vi "niDTS BT Tx Test UTIL Static Default Parameters.vi"(9 "ModulationCharacter Select":T1=enum."BOTH", 10 "BT Standard":T2 caption="802.11 Standard") -> (2 "BT Tx Input Parameters":T3={"Channel"=0, "Data Rate "=1, "Dut Tx Power"=0.0, "External Attenuation (dB)"=[0.0, 0.0, 0.0, 0.0], "Auto Level"=FALSE, "Packet type"=enum."DH1", "Payload Pattern"=enum."PN9", "Burst Sync"=enum."PREamble", "BD ADDRESS"=0, "Packet Length, bytes"=37, "ModAcc Measurement Paramaters"={"ModAcc Enable"=FALSE, "CFO Enable"=FALSE, "Character Select"=enum."DF1", "Averages"=1, "Averaging Mode"=enum."RMS", "Measurement Length"=-1, "Measurement Offset"=0}, "OBW Measurement Parameters"={"OBW Enable"=FALSE, "OBW Averages"=1, "Averaging Type"=enum."RMS", "Measurement Interval Mode"=enum."AUTO", "Measurement Interval Length (sec)"=0.005}, "TXP Measurement Parameters"={"TXP Power Enable"=FALSE, "TXP Averages"=1, "Averaging Type"=enum."RMS"}, "IBE  Measurement Parameters"={"IBE Enable"=FALSE, "IBE Averages"=1, "Averaging Type"=enum."RMS", "Numbe of Channels"=11, "Channel Mode"=enum."Centered", "Measurement Interval Mode"=enum."AUTO", "Measurement Interval Length (sec)"=0.005}, "Trace Enable"=FALSE, "Trigger"={"MinQuietTimeDuration (sec)"=0.0001, "TriggerDelay (sec)"=0.0, "TriggerEdge"=enum."RISing", "TriggerSource"=enum."RF0", "TriggerThreshold (dB)"=-20.0, "TriggerTimeout (sec)"=10.0}} {"BD ADDRESS" max=16777215 format="%.0x"})   [LabVIEW 2015, in "niDTS BT.lvlib"]
uses:
  niDTS BT.lvlib
  Includes/niDTS BT Tx Test INC Parameters.ctl
  Includes/niDTS BT INC Packet Type.ctl
  Includes/niDTS BT Tx Test INC BD Payload Data.ctl
  Includes/niDTS BT Tx Test INC Modulation Characteristics.ctl
  Includes/niDTS BT INC OBW Measurement Parameters.ctl
  Includes/niDTS BT INC TXP Measurement Parameters.ctl
  EDR Tx Test/Includes/niDTS BT INC EDR IBE Measurement Parameters.ctl
  Includes/niDTS BT DUT INC Trigger.ctl
  Includes/niDTS BT INC Standard.ctl
  BDR Tx Test/Includes/niDTS BT BDR Tx Test INC Parameters.ctl
  BDR Tx Test/Includes/niDTS BT INC BDR Packet Type.ctl
  BDR Tx Test/Includes/niDTS BT INC BDR ACP Measurement Parameters.ctl
  EDR Tx Test/Includes/niDTS BT EDR Tx Test INC Parameters.ctl
  EDR Tx Test/Includes/niDTS BT INC EDR Packet Type.ctl
  EDR Tx Test/Includes/niDTS BT INC EDR Data Rate.ctl
  EDR Tx Test/Includes/niDTS BT INC EDR Burst Sync.ctl
  EDR Tx Test/Includes/niDTS BT INC EDR ModAcc Measurement Parameters.ctl
  LE Tx Test/Includes/niDTS BT LE Tx Test INC Parameters.ctl
  LE Tx Test/Includes/niDTS BT INC LE IBE Measurement Parameters.ctl
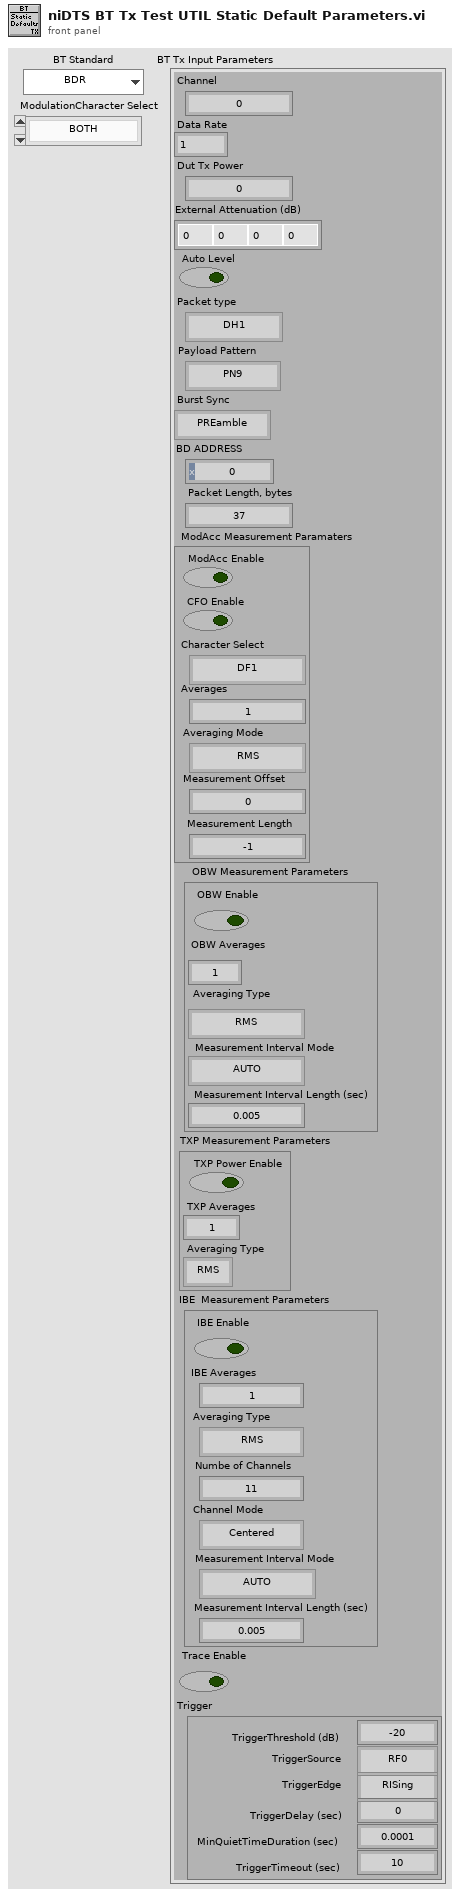
[diagram p1: front panel]
types:
  T1 = typedef "niDTS BT.lvlib/niDTS BT Tx Test INC Modulation Characteristics.ctl" = enum16{"DF1", "DF2", "BOTH"}
  T2 = typedef "niDTS BT.lvlib/niDTS BT INC Standard.ctl" = enum16{"BDR", "EDR", "LE-TP"}
  T3 = typedef "niDTS BT.lvlib/niDTS BT Tx Test INC Parameters.ctl" = cluster{"Channel":i32, "Data Rate ":i32, "Dut Tx Power":dbl, "External Attenuation (dB)":dbl[], "Auto Level":bool, "Packet type":T4, "Payload Pattern":T5, "Burst Sync":enum16{"NONE", "PREamble"}, "BD ADDRESS":u32, "Packet Length, bytes":i32, "ModAcc Measurement Paramaters":cluster{"ModAcc Enable":bool, "CFO Enable":bool, "Character Select":T1, "Averages":i32, "Averaging Mode":enum16{"RMS", "LOG", "SCALAR", "MAX", "MIN", "VECTOR"}, "Measurement Length":i32, "Measurement Offset":i32}, "OBW Measurement Parameters":T6, "TXP Measurement Parameters":T7, "IBE  Measurement Parameters":T8, "Trace Enable":bool, "Trigger":T9}
  T4 = typedef "niDTS BT.lvlib/niDTS BT INC Packet Type.ctl" = enum16{"NULL", "POLL", "FHS", "DM1", "DH1", "HV1", "HV2", "HV3", "EV3", "DV", "AUX1", "DM3", "DH3", "EV4", "EV5", "DM5", "DH5", "LE-TP"}
  T5 = typedef "niDTS BT.lvlib/niDTS BT Tx Test INC BD Payload Data.ctl" = enum16{"0", "1", "01", "00001111", "PN9", "AUTO"}
  T6 = typedef "niDTS BT.lvlib/niDTS BT INC OBW Measurement Parameters.ctl" = cluster{"OBW Enable":bool, "OBW Averages":i32, "Averaging Type":enum16{"RMS", "LOG", "SCALAR", "MAX", "MIN", "VECTOR"}, "Measurement Interval Mode":enum16{"AUTO", "MANUAL"}, "Measurement Interval Length (sec)":dbl}
  T7 = typedef "niDTS BT.lvlib/niDTS BT INC TXP Measurement Parameters.ctl" = cluster{"TXP Power Enable":bool, "TXP Averages":i32, "Averaging Type":enum16{"RMS", "LOG", "SCALAR", "MAX", "MIN"}}
  T8 = typedef "niDTS BT.lvlib/niDTS BT INC EDR IBE Measurement Parameters.ctl" = cluster{"IBE Enable":bool, "IBE Averages":i32, "Averaging Type":enum16{"RMS", "LOG", "SCALAR", "MAX", "MIN", "VECTOR"}, "Numbe of Channels":i32, "Channel Mode":enum16{"InBand", "Centered"}, "Measurement Interval Mode":enum16{"AUTO", "MANUAL"}, "Measurement Interval Length (sec)":dbl}
  T9 = typedef "niDTS BT.lvlib/niDTS BT DUT INC Trigger.ctl" = cluster{"MinQuietTimeDuration (sec)":dbl, "TriggerDelay (sec)":dbl, "TriggerEdge":enum16{"RISing", "FALLing"}, "TriggerSource":enum16{"IMMediate", "RF0", "PFI0", "PFI1", "RTS0", "RTS1", "RTS2", "RTS3", "RTS4", "RTS5", "RTS6", "RTS7", "PXIStar", "SOFT"}, "TriggerThreshold (dB)":dbl, "TriggerTimeout (sec)":dbl}
  T10 = typedef "niDTS BT.lvlib/niDTS BT BDR Tx Test INC Parameters.ctl" = cluster{"Channel":i32, "Dut Tx Power (dBm)":dbl, "Auto Level":bool, "External Attenuation (dB)":dbl, "BDR Packet type":T11, "Payload Data":T5, "Burst Sync":enum16{"NONE", "PREamble"}, "Packet length (bytes)":i32, "BD ADDRESS":string, "Modulation Measurement":cluster{"ModAcc Enable":bool, "CFO Enable":bool, "Character Select":T1, "Averages":i32, "Averaging Mode":enum16{"RMS", "LOG", "SCALAR", "MAX", "MIN", "VECTOR"}, "Measurement Duration (Symbols)":i32, "Measurement Offset (Symbols)":i32}, "Trace Enable":bool, "OBW Measurement":T6, "TXP Measurement":T7, "IBE Measurement":T12, "Trigger":T9}
  T11 = typedef "niDTS BT.lvlib/niDTS BT INC BDR Packet Type.ctl" = enum16{"NULL", "POLL", "FHS", "DM1", "DH1", "HV1", "HV2", "HV3", "EV3", "DV", "AUX1", "DM3", "DH3", "EV4", "EV5", "DM5", "DH5"}
  T12 = typedef "niDTS BT.lvlib/niDTS BT INC BDR ACP Measurement Parameters.ctl" = cluster{"IBE Enable":bool, "IBE Averages":i32, "Averaging Type":enum16{"RMS", "LOG", "SCALAR", "MAX", "MIN", "VECTOR"}, "Numbe of Channels":i32, "Channel Mode":enum16{"InBand", "Centered"}, "Measurement Interval Mode":enum16{"AUTO", "MANUAL"}, "Measurement Interval Length (sec)":dbl}
  T13 = typedef "niDTS BT.lvlib/niDTS BT EDR Tx Test INC Parameters.ctl" = cluster{"Channel":i32, "Dut Tx Power  (dBm)":dbl, "Auto Level":bool, "External Attenuation (dB)":dbl, "EDR Packet type":T14, "Data Rate":T15, "Payload Data":T5, "Burst Sync":T16, "Packet Length, bytes":i32, "BD ADDRESS":string, "Trace Enable":bool, "EDR ModAcc Measurement":T17, "TXP Measurement":T7, "IBE  Measurement":T8, "Trigger":T9}
  T14 = typedef "niDTS BT.lvlib/niDTS BT INC EDR Packet Type.ctl" = enum16{"NULL", "POLL", "FHS", "DM1", "DH1", "HV1", "HV2", "HV3", "EV3", "DV", "AUX1", "DM3", "DH3", "EV4", "EV5", "DM5", "DH5"}
  T15 = typedef "niDTS BT.lvlib/niDTS BT INC EDR Data Rate.ctl" = i32
  T16 = typedef "niDTS BT.lvlib/niDTS BT INC EDR Burst Sync.ctl" = enum16{"NONE", "PREamble"}
  T17 = typedef "niDTS BT.lvlib/niDTS BT INC EDR ModAcc Measurement Parameters.ctl" = cluster{"DEVM Enable":bool, "Averages":i32, "Averaging Mode":enum16{"RMS", "LOG", "SCALAR", "MAX", "MIN", "VECTOR"}, "Measurement Duration (bytes)":i32, "Measurement Offset (bytes)":i32}
  T18 = typedef "niDTS BT.lvlib/niDTS BT LE Tx Test INC Parameters.ctl" = cluster{"Channel":i32, "Dut Tx Power (dBm)":dbl, "Auto Level":bool, "External Attenuation (dB)":dbl, "Payload Data":T5, "Burst Sync":enum16{"NONE", "PREamble"}, "Packet Length (bytes)":i32, "Modulation Measurement":cluster{"ModAcc Enable":bool, "CFO Enable":bool, "Character Select":T1, "Averages":i32, "Averaging Mode":enum16{"RMS", "LOG", "SCALAR", "MAX", "MIN", "VECTOR"}, "Measurement Duration (bytes)":i32, "Measurement Offset (bytes)":i32}, "TXP Measurement":T7, "LE IBE Measurement":T19, "Trace Enable":bool, "Trigger":T9}
  T19 = typedef "niDTS BT.lvlib/niDTS BT INC LE IBE Measurement Parameters.ctl" = cluster{"LE IBE Enable":bool, "LE IBE Averages":i32, "Averaging Type":enum16{"RMS", "LOG", "SCALAR", "MAX", "MIN", "VECTOR"}, "Numbe of Channels":i32, "Channel Mode":enum16{"InBand", "Centered"}, "Measurement Interval Mode":enum16{"AUTO", "MANUAL"}, "Measurement Interval Length (sec)":dbl}
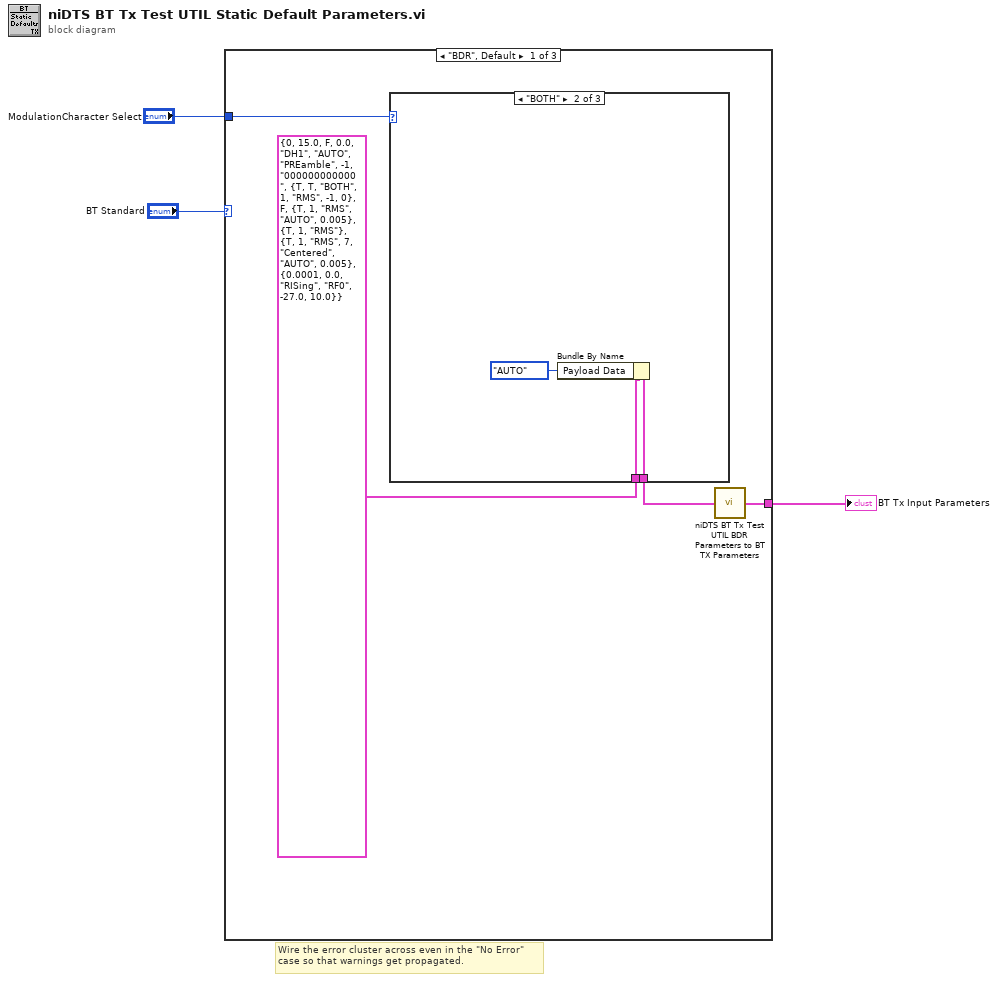
[diagram p0: block diagram]
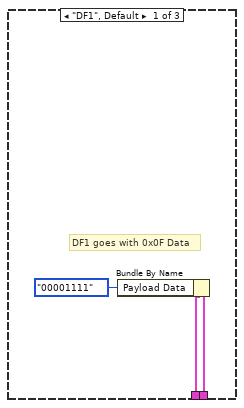
[diagram p2: hidden frame]
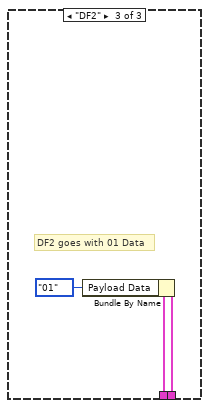
[diagram p3: hidden frame]
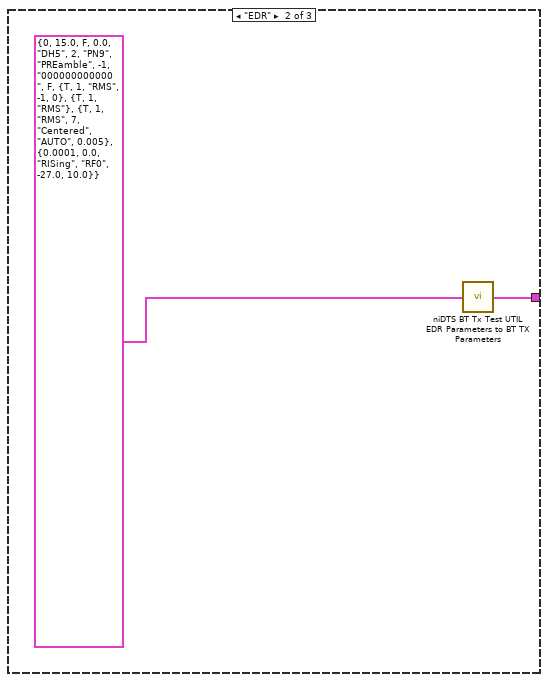
[diagram p4: hidden frame]
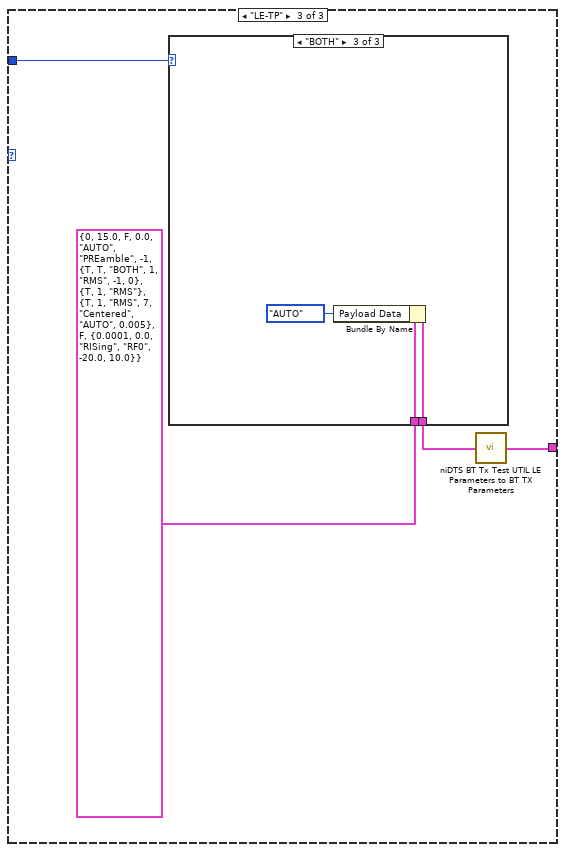
[diagram p5: hidden frame]
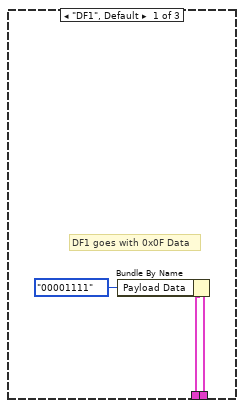
[diagram p6: hidden frame]
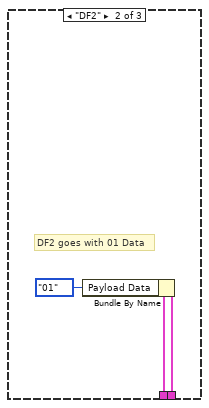
[diagram p7: hidden frame]
diagram:
  # "Wire the error cluster across even in the \"No Error\"\ncase so that warnings get propagated."
  n1 = case shown="\"BDR\", Default" "BT Standard" {
    tunnel: [w7 w18 w22] -> w2
    tunnel: "ModulationCharacter Select" -> [w4 _ w21]
    frame "BDR", Default {
      n2 = case shown="\"BOTH\"" w4 {
        tunnel: T10 {"Channel"=0, "Dut Tx Power (dBm)"=15.0, "Auto Level"=FALSE, "External Attenuation (dB)"=0.0, "BDR Packet type"=enum."DH1", "Payload Data"=enum."AUTO", "Burst Sync"=enum."PREamble", "Packet length (bytes)"=-1, "BD ADDRESS"="000000000000 ", "Modulation Measurement"={"ModAcc Enable"=TRUE, "CFO Enable"=TRUE, "Character Select"=enum."BOTH", "Averages"=1, "Averaging Mode"=enum."RMS", "Measurement Duration (Symbols)"=-1, "Measurement Offset (Symbols)"=0}, "Trace Enable"=FALSE, "OBW Measurement"={"OBW Enable"=TRUE, "OBW Averages"=1, "Averaging Type"=enum."RMS", "Measurement Interval Mode"=enum."AUTO", "Measurement Interval Length (sec)"=0.005}, "TXP Measurement"={"TXP Power Enable"=TRUE, "TXP Averages"=1, "Averaging Type"=enum."RMS"}, "IBE Measurement"={"IBE Enable"=TRUE, "IBE Averages"=1, "Averaging Type"=enum."RMS", "Numbe of Channels"=7, "Channel Mode"=enum."Centered", "Measurement Interval Mode"=enum."AUTO", "Measurement Interval Length (sec)"=0.005}, "Trigger"={"MinQuietTimeDuration (sec)"=0.0001, "TriggerDelay (sec)"=0.0, "TriggerEdge"=enum."RISing", "TriggerSource"=enum."RF0", "TriggerThreshold (dB)"=-27.0, "TriggerTimeout (sec)"=10.0}} ("BDR Tx Input Parameters") -> [w9 w12 w16]
        tunnel: [w8 w11 w15] -> w5
        frame "DF1", Default {
          # "DF1 goes with 0x0F Data"
          n3 = Bundle By Name(cluster=w9, "Payload Data"=niDTS_BT_Tx_Test_INC_BD_Payload_Data."00001111") -> (w8:T10)
        }
        frame "BOTH" {
          n4 = Bundle By Name(cluster=w12, "Payload Data"=niDTS_BT_Tx_Test_INC_BD_Payload_Data."AUTO") -> (w11:T10)
        }
        frame "DF2" {
          # "DF2 goes with 01 Data"
          n5 = Bundle By Name(cluster=w16, "Payload Data"=niDTS_BT_Tx_Test_INC_BD_Payload_Data."01") -> (w15:T10)
        }
      }
      n6 = call "niDTS BT Tx Test UTIL BDR Parameters to BT TX Parameters.vi"("BT BDR Parameters"=w5) -> ("BT Tx Parameters"=w7:T3)  [unwired: 14 in]
    }
    frame "EDR" {
      n7 = call "niDTS BT Tx Test UTIL EDR Parameters to BT TX Parameters.vi"("EDR Tx Input Parameters"=T13 {"Channel"=0, "Dut Tx Power  (dBm)"=15.0, "Auto Level"=FALSE, "External Attenuation (dB)"=0.0, "EDR Packet type"=enum."DH5", "Data Rate"=2, "Payload Data"=enum."PN9", "Burst Sync"=enum."PREamble", "Packet Length, bytes"=-1, "BD ADDRESS"="000000000000 ", "Trace Enable"=FALSE, "EDR ModAcc Measurement"={"DEVM Enable"=TRUE, "Averages"=1, "Averaging Mode"=enum."RMS", "Measurement Duration (bytes)"=-1, "Measurement Offset (bytes)"=0}, "TXP Measurement"={"TXP Power Enable"=TRUE, "TXP Averages"=1, "Averaging Type"=enum."RMS"}, "IBE  Measurement"={"IBE Enable"=TRUE, "IBE Averages"=1, "Averaging Type"=enum."RMS", "Numbe of Channels"=7, "Channel Mode"=enum."Centered", "Measurement Interval Mode"=enum."AUTO", "Measurement Interval Length (sec)"=0.005}, "Trigger"={"MinQuietTimeDuration (sec)"=0.0001, "TriggerDelay (sec)"=0.0, "TriggerEdge"=enum."RISing", "TriggerSource"=enum."RF0", "TriggerThreshold (dB)"=-27.0, "TriggerTimeout (sec)"=10.0}}) -> ("BT Tx Input Parameters"=w18:T3)  [unwired: 14 in]
    }
    frame "LE-TP" {
      n8 = case shown="\"BOTH\"" w21 {
        tunnel: T18 {"Channel"=0, "Dut Tx Power (dBm)"=15.0, "Auto Level"=FALSE, "External Attenuation (dB)"=0.0, "Payload Data"=enum."AUTO", "Burst Sync"=enum."PREamble", "Packet Length (bytes)"=-1, "Modulation Measurement"={"ModAcc Enable"=TRUE, "CFO Enable"=TRUE, "Character Select"=enum."BOTH", "Averages"=1, "Averaging Mode"=enum."RMS", "Measurement Duration (bytes)"=-1, "Measurement Offset (bytes)"=0}, "TXP Measurement"={"TXP Power Enable"=TRUE, "TXP Averages"=1, "Averaging Type"=enum."RMS"}, "LE IBE Measurement"={"LE IBE Enable"=TRUE, "LE IBE Averages"=1, "Averaging Type"=enum."RMS", "Numbe of Channels"=7, "Channel Mode"=enum."Centered", "Measurement Interval Mode"=enum."AUTO", "Measurement Interval Length (sec)"=0.005}, "Trace Enable"=FALSE, "Trigger"={"MinQuietTimeDuration (sec)"=0.0001, "TriggerDelay (sec)"=0.0, "TriggerEdge"=enum."RISing", "TriggerSource"=enum."RF0", "TriggerThreshold (dB)"=-20.0, "TriggerTimeout (sec)"=10.0}} ("LE Tx Input Parameters") -> [w24 w28 w31]
        tunnel: [w23 w27 w30] -> w19
        frame "DF1", Default {
          # "DF1 goes with 0x0F Data"
          n9 = Bundle By Name(cluster=w24, "Payload Data"=niDTS_BT_Tx_Test_INC_BD_Payload_Data."00001111") -> (w23:T18)
        }
        frame "DF2" {
          # "DF2 goes with 01 Data"
          n10 = Bundle By Name(cluster=w28, "Payload Data"=niDTS_BT_Tx_Test_INC_BD_Payload_Data."01") -> (w27:T18)
        }
        frame "BOTH" {
          n11 = Bundle By Name(cluster=w31, "Payload Data"=niDTS_BT_Tx_Test_INC_BD_Payload_Data."AUTO") -> (w30:T18)
        }
      }
      n12 = call "niDTS BT Tx Test UTIL LE Parameters to BT TX Parameters.vi"("LE Tx Input Parameters"=w19) -> ("BT Tx Parameters"=w22:T3)  [unwired: 14 in]
    }
  }
  "BT Tx Input Parameters" <- w2
